vi "Decode boolean.vi"(8 "error in (no error)":errorcluster, 11 "Data":variant) -> (0 "error out":errorcluster, 3 "Boolean":bool)   [LabVIEW 2026, in "TALOS.lvlib" / "Guardian.lvlib" / "Guardian.lvclass"]
uses:
  Guardian.lvclass
  TALOS.lvlib
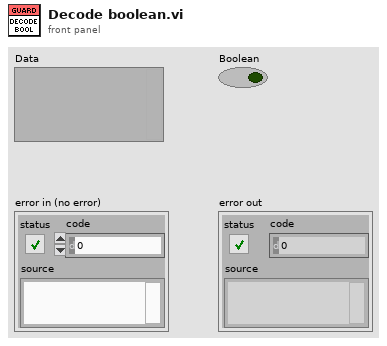
[diagram p1: front panel]
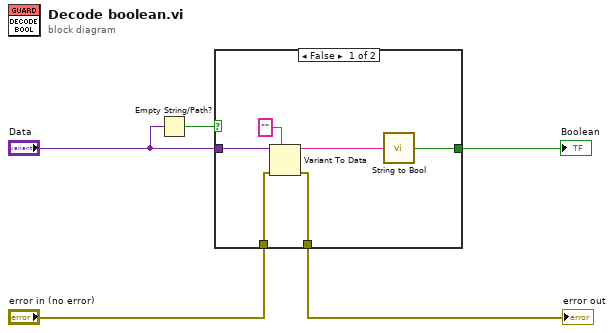
[diagram p0: block diagram]
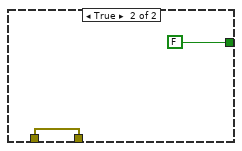
[diagram p2: hidden frame]
diagram:
  n1 = Empty String/Path?(string/path="Data") -> (empty?=w1:bool)
  n2 = case shown="False" w1 {
    tunnel: [w11 FALSE ("Boolean")] -> w5
    tunnel: "error in (no error)" -> [w10 w12]
    tunnel: [w9 w12] -> w3
    tunnel: "Data" -> [w6 _]
    frame False {
      n3 = Variant To Data(error in=w10, type="", Variant=w6) -> (data=w8:string, error out=w9:errorcluster)
      n4 = call "String to Bool.vi"("String"=w8) -> ("Boolean"=w11:bool)
    }
    frame True {
    }
  }
  "Boolean" <- w5
  "error out" <- w3
